vi "Divide.vi"(1 "x":sgl, 2 "y":sgl, 4 "Divider":refnum<class "Divider.lvclass">) -> (6 "x/y":sgl)   [LabVIEW 2017, in "Divider.lvclass"]
uses:
  Divider.lvclass
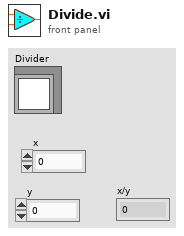
[diagram p1: front panel]
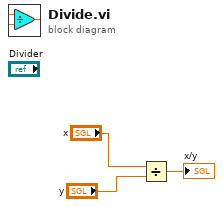
[diagram p0: block diagram]
diagram:
  n1 = Divide(x="x", y="y") -> (x/y=→"x/y":sgl)
